vi "chart.vi"() -> ()   [LabVIEW 2017]
panel:
  out "Waveform Chart":cluster{"Температура":dbl, dbl, dbl}(graph)
  out "random num":dbl
  out "average":dbl
  in  "stop":bool
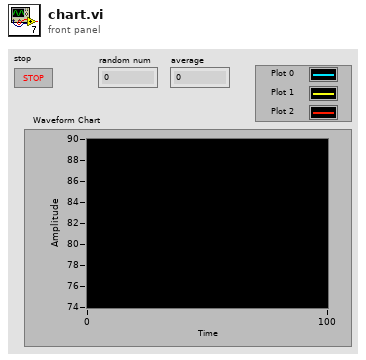
[diagram p1: front panel]
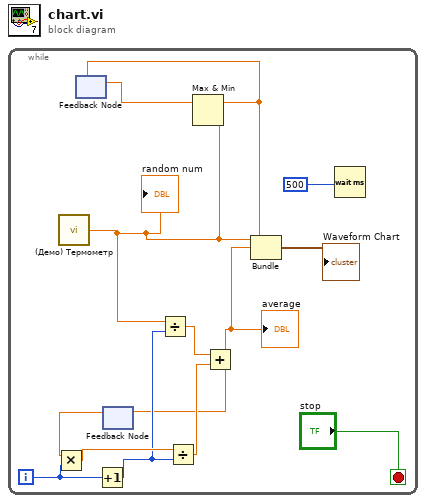
[diagram p0: block diagram]
diagram:
  n1 = while {
    i -> [w10]
    stop <- "stop" stop-if-true
    n2 = call "(Демо) Термометр.vi"() -> ("Температура"=w2:dbl)  [unwired: 1 in]
    "random num" <- w2
    n3 = feedback #1() -> (w3:dbl)  [unwired: 1 in]
    n4 = Increment(x=w10) -> (x+1=w6:i32)
    n5 = feedback #2() -> (w11:dbl)  [unwired: 1 in]
    n6 = Multiply(x=w11, y=w10) -> (x*y=w9:dbl)
    n7 = Divide(x=w2, y=w6) -> (x/y=w12:dbl)
    n8 = Divide(x=w9, y=w6) -> (x/y=w7:dbl)
    n9 = Max & Min(x=w3, y=w2) -> (max(x,y)=w1:dbl)  [unwired: 1 out]
    n10 = feedback-in #1(w1) -> ()
    n11 = Add(x=w12, y=w7) -> (x+y=w5:dbl)
    "average" <- w5
    n12 = feedback-in #2(w5) -> ()
    n13 = Bundle("Температура"=w2, w5, w1) -> (→"Waveform Chart":cluster{"Температура":dbl, dbl, dbl})  [unwired: 1 in]
    n14 = Wait (ms)(milliseconds to wait=500) -> ()  [unwired: 1 out]
  }
